vi "Write String Refnum.vi"(8 "error in (no error)":errorcluster, 10 "String Refnum":refnum<vi>, 11 "String Control in":refnum<class "String Control.lvclass">) -> (0 "error out":errorcluster, 3 "String Control out":refnum<class "String Control.lvclass">)   [LabVIEW 2010, in "String Control.lvclass"]
uses:
  String Control.lvclass
  String Control.lvclass/String Control.ctl
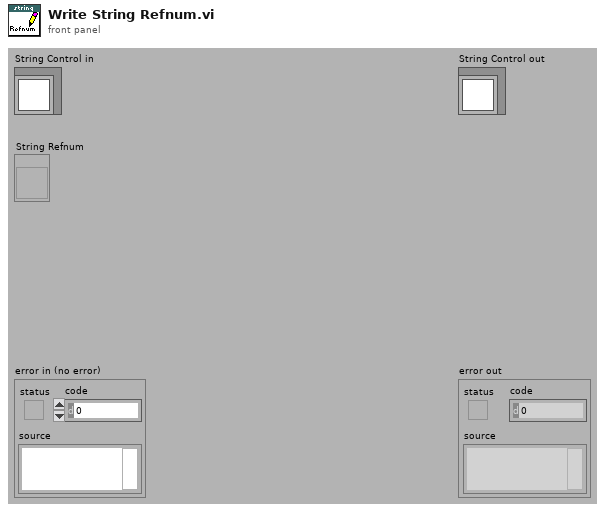
[diagram p1: front panel]
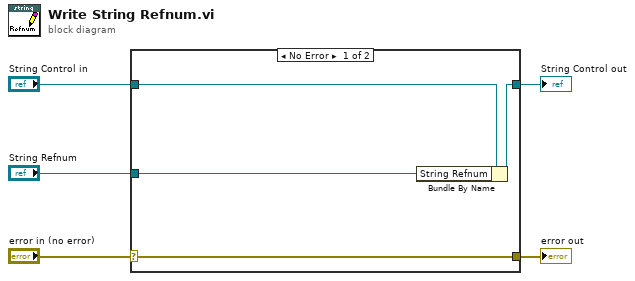
[diagram p0: block diagram]
diagram:
  n1 = case shown="No Error" "error in (no error)" {
    selector: "error in (no error)" -> [w9 w10]
    tunnel: [w9 w10] -> w4
    tunnel: [w7 w11] -> w2
    tunnel: "String Control in" -> [w8 w11]
    tunnel: "String Refnum" -> [w6 _]
    frame No Error {
      n2 = Bundle By Name(cluster=w8, "String Refnum"=w6) -> (w7:refnum<class "String Control.lvclass">)
    }
    frame Error {
    }
  }
  "error out" <- w4
  "String Control out" <- w2
